vi "connect channel to tag.vi"(7 "Tag Enum In":i32, 8 "error in (no error)":errorcluster, 9 "UID":string, 10 "TBM channel in":refnum<class "TBM channel.lvclass">, 11 "engine configuration in":refnum<class "engine configuration.lvclass">) -> (0 "error out":errorcluster, 3 "engine configuration out":refnum<class "engine configuration.lvclass">)   [LabVIEW 2014]
uses:
  <vilib>/NI/Module Execution Interface/Engine Configuration/engine configuration.lvclass
  <vilib>/NI/Tag Bus Module Framework/channel/TBM channel.lvclass
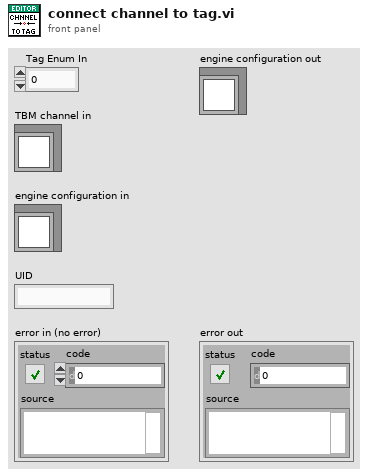
[diagram p1: front panel]
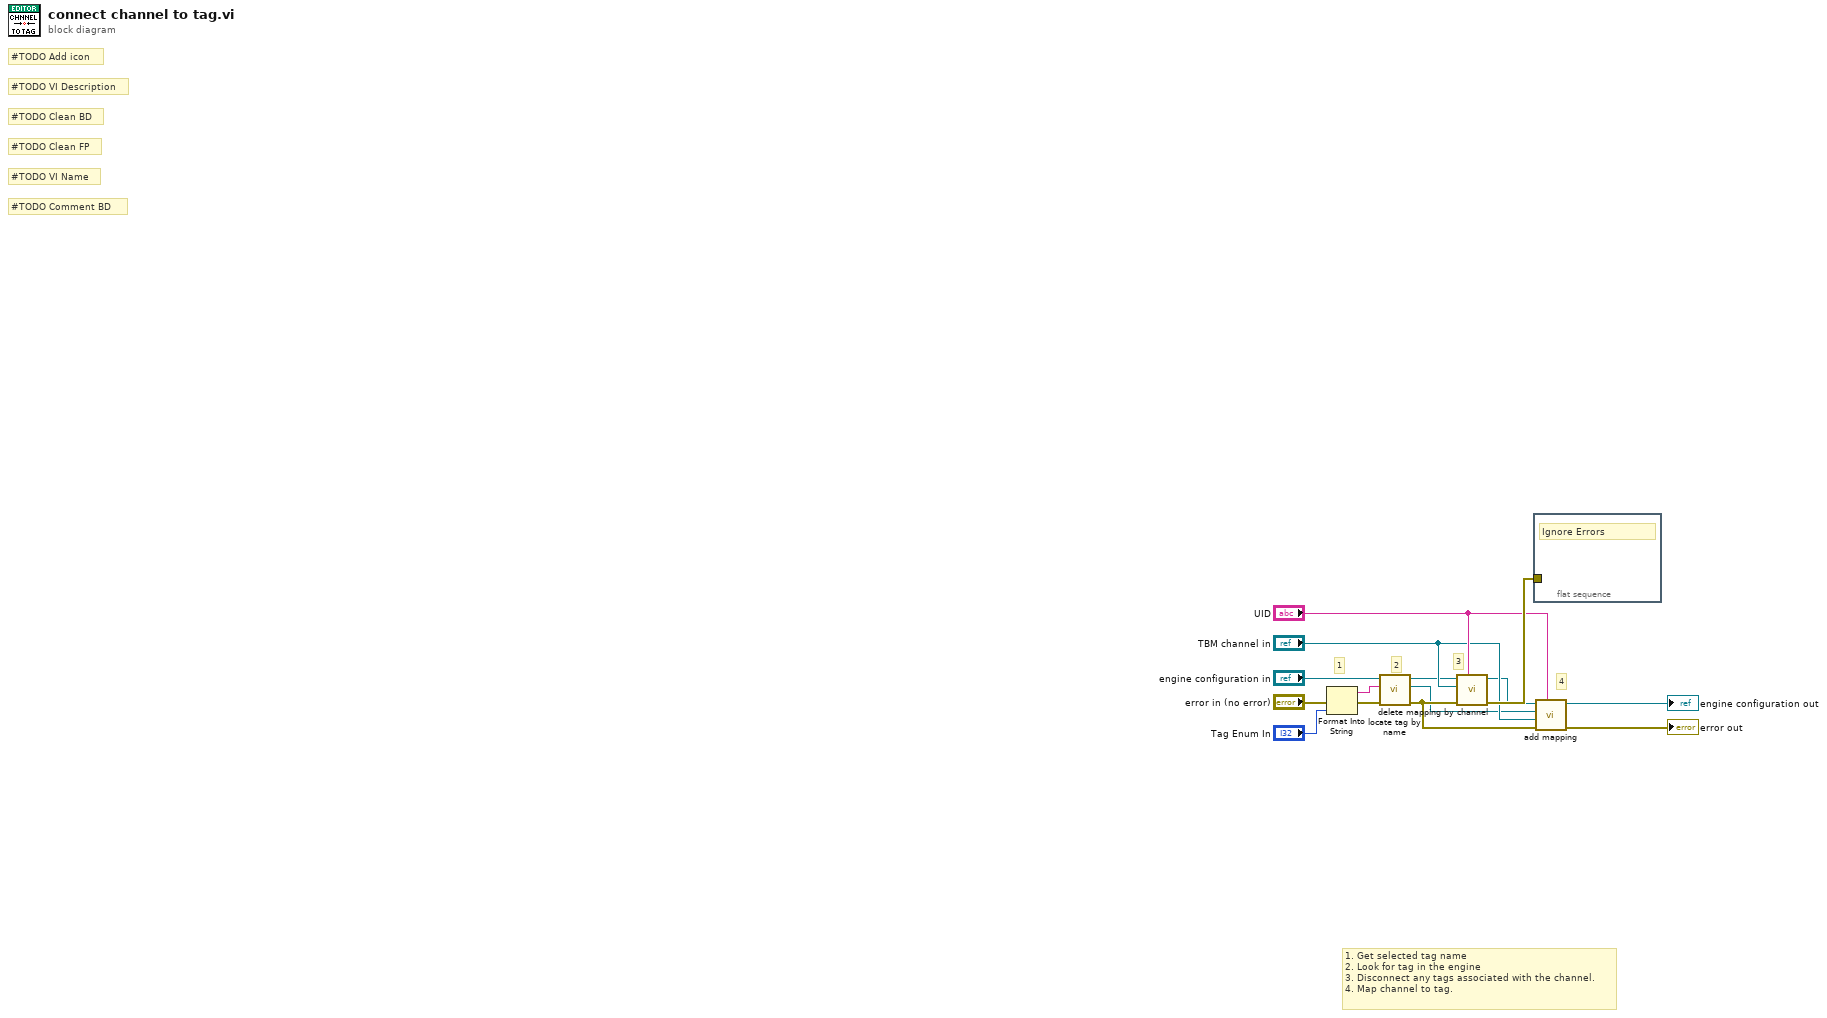
[diagram p0: block diagram]
diagram:
  # "#TODO Comment BD"
  # "#TODO VI Name"
  # "#TODO Clean FP"
  # "#TODO Clean BD"
  # "#TODO VI Description"
  # "#TODO Add icon"
  # "1. Get selected tag name\n2. Look for tag in the engine\n3. Disconnect any tags associated with the channel.\n4. Map channel to tag."
  # "4"
  # "3"
  # "2"
  # "1"
  n1 = Format Into String(error in="error in (no error)", "Tag Enum In") -> (resulting string=w3:string, error out=w13:errorcluster)  [unwired: 2 in]
  n2 = call <vilib>:"locate tag by name.vi"("error in"=w13, "tag name"=w3, "engine configuration in"="engine configuration in") -> ("error out"=w10:errorcluster, "tag descriptor"=w6:refnum<class "tag descriptor.lvclass">, "engine configuration out"=w4:refnum<class "engine configuration.lvclass">)  [unwired: 6 in]
  n3 = call <vilib>:"delete mapping by channel.vi"("owner ID"="UID", "error in"=w10, "channel"="TBM channel in", "engine configuration in"=w4) -> ("error out"=w11:errorcluster, "engine configuration out"=w5:refnum<class "engine configuration.lvclass">)  [unwired: 6 in]
  n4 = flat-sequence {
    tunnel: w11 -> [_]
    frame #0 {
      # "Ignore Errors"
    }
  }
  n5 = call <vilib>:"add mapping.vi"("owner ID"="UID", "error in"=w10, "channel"="TBM channel in", "tag descriptor"=w6, "engine configuration"=w5) -> ("error out"=→"error out":errorcluster, "engine configuration out"=→"engine configuration out":refnum<class "engine configuration.lvclass">)  [unwired: 5 in]
